vi "Image AE.vi"(7 "Image State":T1, 8 "Pane Color":u32, 9 "Header Path":path, 10 "Images":T2[](array[typedef]), 11 "Path":path=path "C:/Users/telsey/Desktop/Personal Projects/Photobooth/Photos") -> (3 "New Image Path":path)   [LabVIEW 2012]
uses:
  <vilib>/vision/Image Controls.llb/IMAQ Image.ctl
  Image States.ctl
panel:
  out "Image 4":T2(plugin-control)
  out "Image 2":T2(plugin-control)
  out "Image 3":T2(plugin-control)
  out "Image":T2(plugin-control)
  out "Header":picture
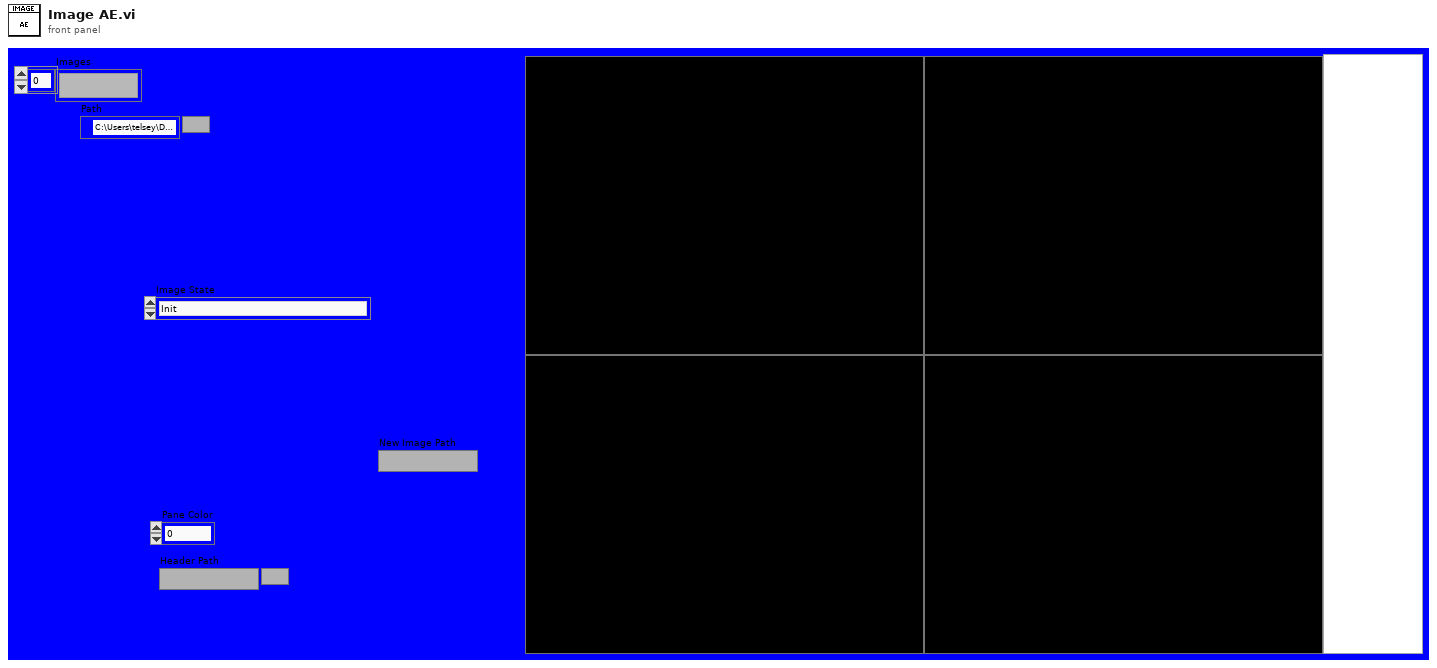
[diagram p1: front panel]
types:
  T1 = typedef "Image States.ctl" = enum16{"Init", "Print"}
  T2 = typedef "IMAQ Image.ctl" = refnum<image>
  T3 = typedef "imagedata.ctl" = cluster{"image type":i32, "image depth":i32, "image":u8[], "mask":u8[], "colors":u32[], "Rectangle":cluster{"left":i16, "top":i16, "right":i16, "bottom":i16}}
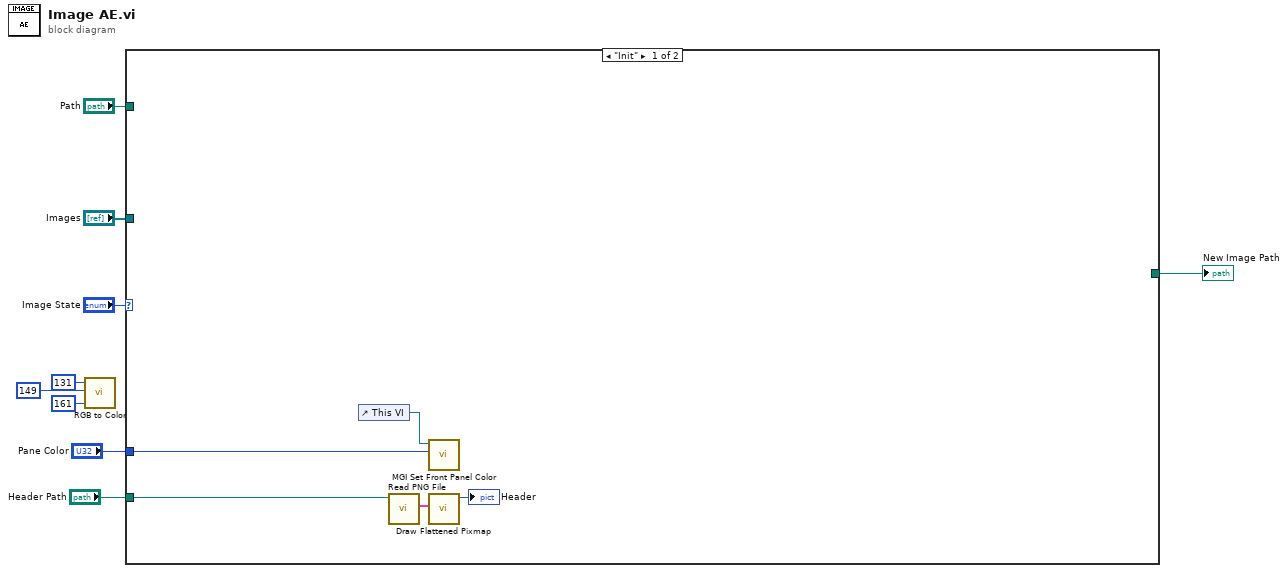
[diagram p0: block diagram]
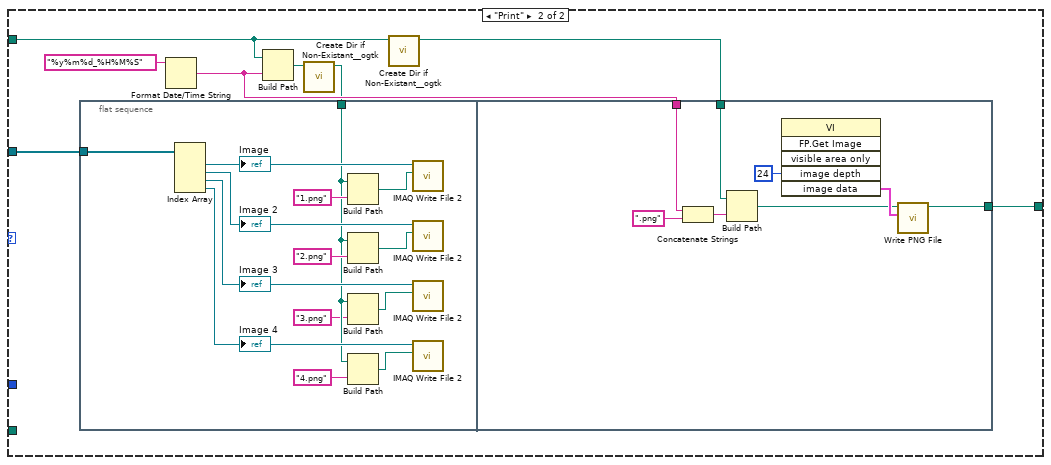
[diagram p2: hidden frame]
diagram:
  n1 = call <vilib>:"RGB to Color.vi"("B"=u8 161, "G"=u8 149, "R"=u8 131) -> ()  [unwired: 1 out]
  n2 = case shown="\"Init\"" "Image State" {
    tunnel: "Path" -> [_ w18]
    tunnel: "Images" -> [_ w16]
    tunnel: [_ w15] -> w7
    tunnel: "Pane Color" -> [w10 _]
    tunnel: "Header Path" -> [w14 _]
    frame "Init" {
      n3 = control-ref of="This VI"() -> (w11:refnum<vi>)
      n4 = call <vilib>:"Read PNG File.vi"("path to PNG file"=w14) -> ("image data"=w13:T3)  [unwired: 8 in, 2 out]
      n5 = call <userlib>:"MGI Set Front Panel Color.vi"("Color (System Panel)"=w10, "VI Reference In (Caller)"=w11) -> ()  [unwired: 7 in, 2 out]
      n6 = call <vilib>:"Draw Flattened Pixmap.vi"("image data"=w13) -> ("new picture"=→"Header":picture)  [unwired: 8 in]
    }
    frame "Print" {
      n7 = flat-sequence {
        tunnel: w19 -> [w26]
        tunnel: w16 -> [w23]
        tunnel: w21 -> [w41]
        tunnel: w17 -> [w39]
        tunnel: [w37] -> w15
        frame #0 {
          n8 = Index Array(array=w23) -> (element #1=w33:T2, element #2=w34:T2, element #3=w35:T2, element #4=w36:T2)  [unwired: 4 in]
          "Image" <- w33
          "Image 2" <- w34
          "Image 3" <- w35
          "Image 4" <- w36
          n9 = Build Path(base path=w26, name or relative path="1.png") -> (appended path=w32:path)
          n10 = Build Path(base path=w26, name or relative path="2.png") -> (appended path=w31:path)
          n11 = Build Path(base path=w26, name or relative path="3.png") -> (appended path=w30:path)
          n12 = Build Path(base path=w26, name or relative path="4.png") -> (appended path=w29:path)
          n13 = call-poly "IMAQ Write File 2"("File Path"=w32, "Image"=w33) -> ()  [unwired: 8 in, 2 out]
          n14 = call-poly "IMAQ Write File 2"("File Path"=w31, "Image"=w34) -> ()  [unwired: 8 in, 2 out]
          n15 = call-poly "IMAQ Write File 2"("File Path"=w30, "Image"=w35) -> ()  [unwired: 8 in, 2 out]
          n16 = call-poly "IMAQ Write File 2"("File Path"=w29, "Image"=w36) -> ()  [unwired: 8 in, 2 out]
        }
        frame #1 {
          n17 = Concatenate Strings(w41, ".png" ("string")) -> (w40:string)
          n18 = Build Path(base path=w39, name or relative path=w40) -> (appended path=w38:path)
          n19 = invoke class="VI" method="FP.Get Image"("image depth"=24 ("Image Depth")) -> ("image data"=w42:T3)  [unwired: 5 in, 5 out]
          n20 = call <vilib>:"Write PNG File.vi"("image data"=w42, "path to PNG file"=w38) -> ("path"=w37:path)  [unwired: 8 in, 1 out]
        }
      }
      n21 = Format Date/Time String(time format string (%c)="%y%m%d_%H%M%S") -> (date/time string=w21:string)  [unwired: 2 in]
      n22 = Build Path(base path=w18, name or relative path=w21) -> (appended path=w20:path)
      n23 = call <userlib>:"Create Dir if Non-Existant__ogtk.vi"("Directory Path"=w20) -> ("dup Directory Path"=w19:path)  [unwired: 8 in, 2 out]
      n24 = call <userlib>:"Create Dir if Non-Existant__ogtk.vi"("Directory Path"=w18) -> ("dup Directory Path"=w17:path)  [unwired: 8 in, 2 out]
    }
  }
  "New Image Path" <- w7
